vi "cumplimiento_ext.vi"(8 "error in (no error)":errorcluster, 11 "Prueba08 in":refnum<class "Prueba031.lvclass">) -> (0 "error out":errorcluster, 2 "cumpimiento":string, 3 "Prueba08 out":refnum<class "Prueba031.lvclass">)   [LabVIEW 2019, in "Prueba031.lvclass"]
uses:
  Prueba031.lvclass
  Prueba031.lvclass/Prueba031.ctl
  RerenceAllControlsToolkit/_get control reference by name.vi
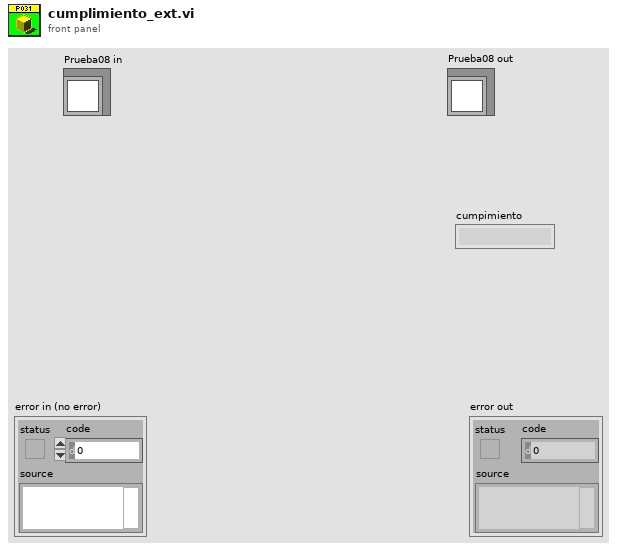
[diagram p1: front panel]
types:
  T1 = cluster{"Medido":dbl, "Medido_Cor":dbl, "Error":dbl, "Ref":dbl, "Incert_exp":dbl, "Tol+":dbl, "Tol-":dbl, "fila":i32}
  T2 = cluster{"ControlName":string, "ControlReference":refnum<vi>}[]
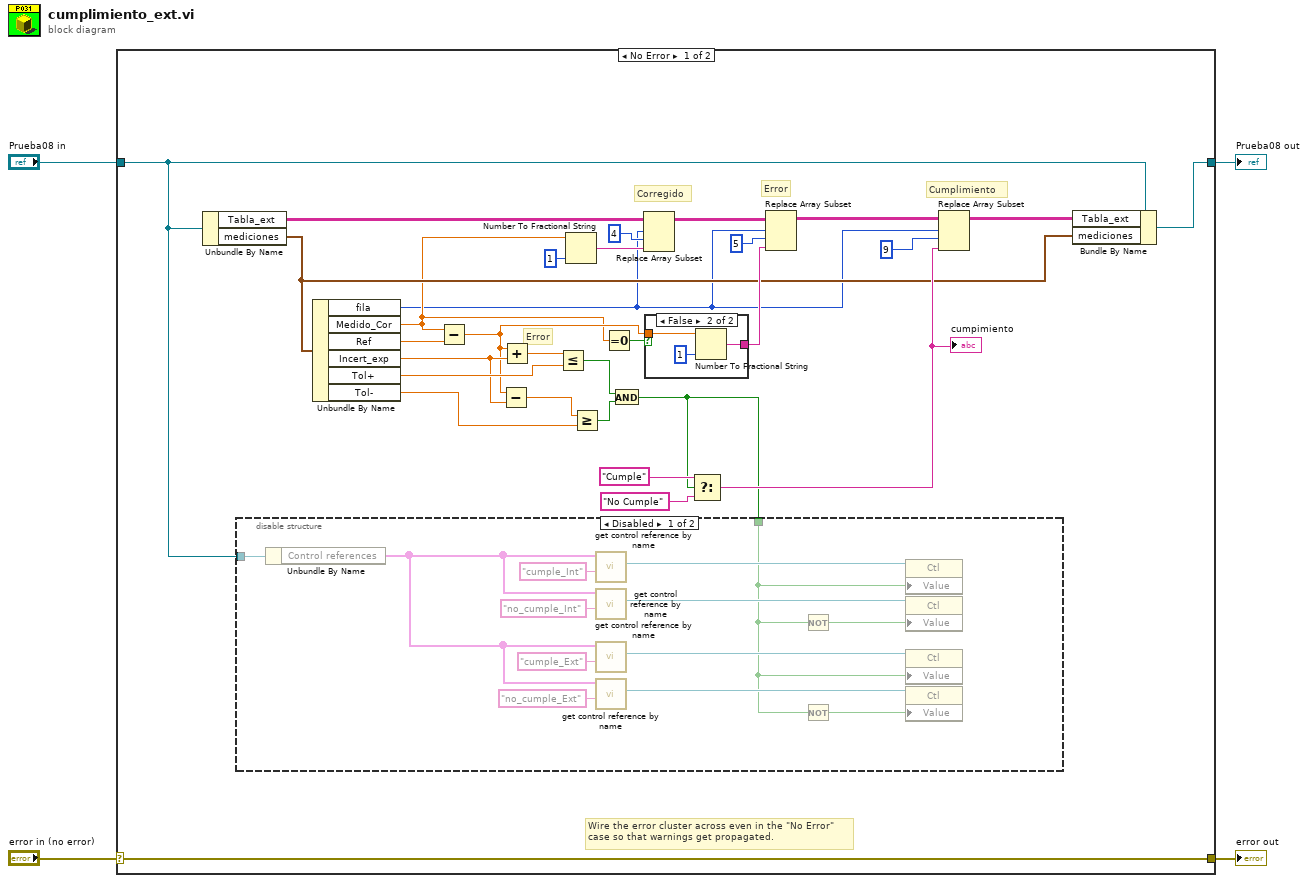
[diagram p0: block diagram]
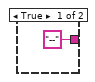
[diagram p3: hidden frame]
diagram:
  n1 = case shown="No Error" "error in (no error)" {
    selector: "error in (no error)" -> [w34 w53]
    tunnel: [w34 w53] -> w3
    tunnel: [w16 w52] -> w2
    tunnel: "Prueba08 in" -> [w12 w52]
    frame No Error {
      # "Corregido"
      # "Cumplimiento"
      # "Error"
      # "Error"
      # "Wire the error cluster across even in the \"No Error\"\ncase so that warnings get propagated."
      n2 = Unbundle By Name(w12) -> ("Tabla_ext"=w14:string[][], "mediciones"=w13:T1)
      n3 = Unbundle By Name(w13) -> ("fila"=w5:i32, "Medido_Cor"=w8:dbl, "Ref"=w27:dbl, "Incert_exp"=w25:dbl, "Tol+"=w26:dbl, "Tol-"=w24:dbl)
      n4 = Subtract(x=w8, y=w27) -> (x-y=w17:dbl)
      n5 = Subtract(x=w17, y=w25) -> (x-y=w30:dbl)
      n6 = Add(x=w17, y=w25) -> (x+y=w33:dbl)
      n7 = Less Or Equal?(x=w33, y=w26) -> (x <= y?=w32:bool)
      n8 = Number To Fractional String(number=w8, precision (6)=i16 1) -> (F-format string=w7:string)  [unwired: 2 in]
      n9 = Greater Or Equal?(x=w30, y=w24) -> (x >= y?=w31:bool)
      n10 = Equal To 0?(x=w8) -> (x = 0?=w18:bool)
      n11 = And(x=w32, y=w31) -> (x .and. y?=w11:bool)
      n12 = disable-structure shown="Disabled" {
        disable-tunnel: w12 -> [w47 _]
        disable-tunnel: w11 -> [w35 _]
        frame Disabled {
          n13 = Unbundle By Name(w47) -> ("Control references"=w36:T2)
          n14 = call-poly "get control reference by name.vi"("Control name"="cumple_Int", "Control references"=w36) -> ("Ctl Refnum"=w46:refnum<vi>)  [unwired: 4 in, 1 out]
          n15 = call-poly "get control reference by name.vi"("Control name"="no_cumple_Int", "Control references"=w36) -> ("Ctl Refnum"=w43:refnum<vi>)  [unwired: 4 in, 1 out]
          n16 = call-poly "get control reference by name.vi"("Control name"="cumple_Ext", "Control references"=w36) -> ("Ctl Refnum"=w37:refnum<vi>)  [unwired: 4 in, 1 out]
          n17 = call-poly "get control reference by name.vi"("Control name"="no_cumple_Ext", "Control references"=w36) -> ("Ctl Refnum"=w40:refnum<vi>)  [unwired: 4 in, 1 out]
          n18 = Not(x=w35) -> (.not. x?=w42:bool)
          n19 = Not(x=w35) -> (.not. x?=w41:bool)
          n20 = property class="Ctl"(reference=w46, "Value"=w35) -> ()  [unwired: 1 in, 2 out]
          n21 = property class="Ctl"(reference=w43, "Value"=w42) -> ()  [unwired: 1 in, 2 out]
          n22 = property class="Ctl"(reference=w37, "Value"=w35) -> ()  [unwired: 1 in, 2 out]
          n23 = property class="Ctl"(reference=w40, "Value"=w41) -> ()  [unwired: 1 in, 2 out]
        }
        frame Enabled {
        }
      }
      n24 = Replace Array Subset(array=w14, new element=w7, index (row)=w5, index (col)=4 ("disabled index (col)")) -> (w10:string[][])
      n25 = case shown="False" w18 {
        tunnel: w17 -> [_ w51]
        tunnel: ["--" w49] -> w19
        frame True {
        }
        frame False {
          n26 = Number To Fractional String(number=w51, precision (6)=i16 1) -> (F-format string=w49:string)  [unwired: 2 in]
        }
      }
      n27 = Select(t="Cumple", s=w11, f="No Cumple") -> (s? t:f=w23:string)
      "cumpimiento" <- w23
      n28 = Replace Array Subset(array=w10, new element=w19, index (row)=w5, index (col)=5 ("disabled index (col)")) -> (w21:string[][])
      n29 = Replace Array Subset(array=w21, new element=w23, index (row)=w5, index (col)=9 ("index (row)")) -> (w15:string[][])
      n30 = Bundle By Name(cluster=w12, "Tabla_ext"=w15, "mediciones"=w13) -> (w16:refnum<class "Prueba031.lvclass">)
    }
    frame Error {
    }
  }
  "error out" <- w3
  "Prueba08 out" <- w2
